vi "Find Intersecting Gaps.vi"(10 "Job Gaps Array":i32[][](array[numeric]), 11 "Machine Gaps Array":i32[][](array[numeric])) -> (3 "Gaps Array":T1[](array[typedef]))   [LabVIEW 2013, in "Scheduler.lvclass"]
uses:
  Scheduler.lvclass
  Controls/ValidGaps.ctl
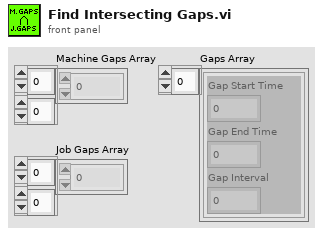
[diagram p1: front panel]
types:
  T1 = typedef "Scheduler.lvclass/ValidGaps.ctl" = cluster{"Gap Start Time":i32, "Gap End Time":i32, "Gap Interval":i32}
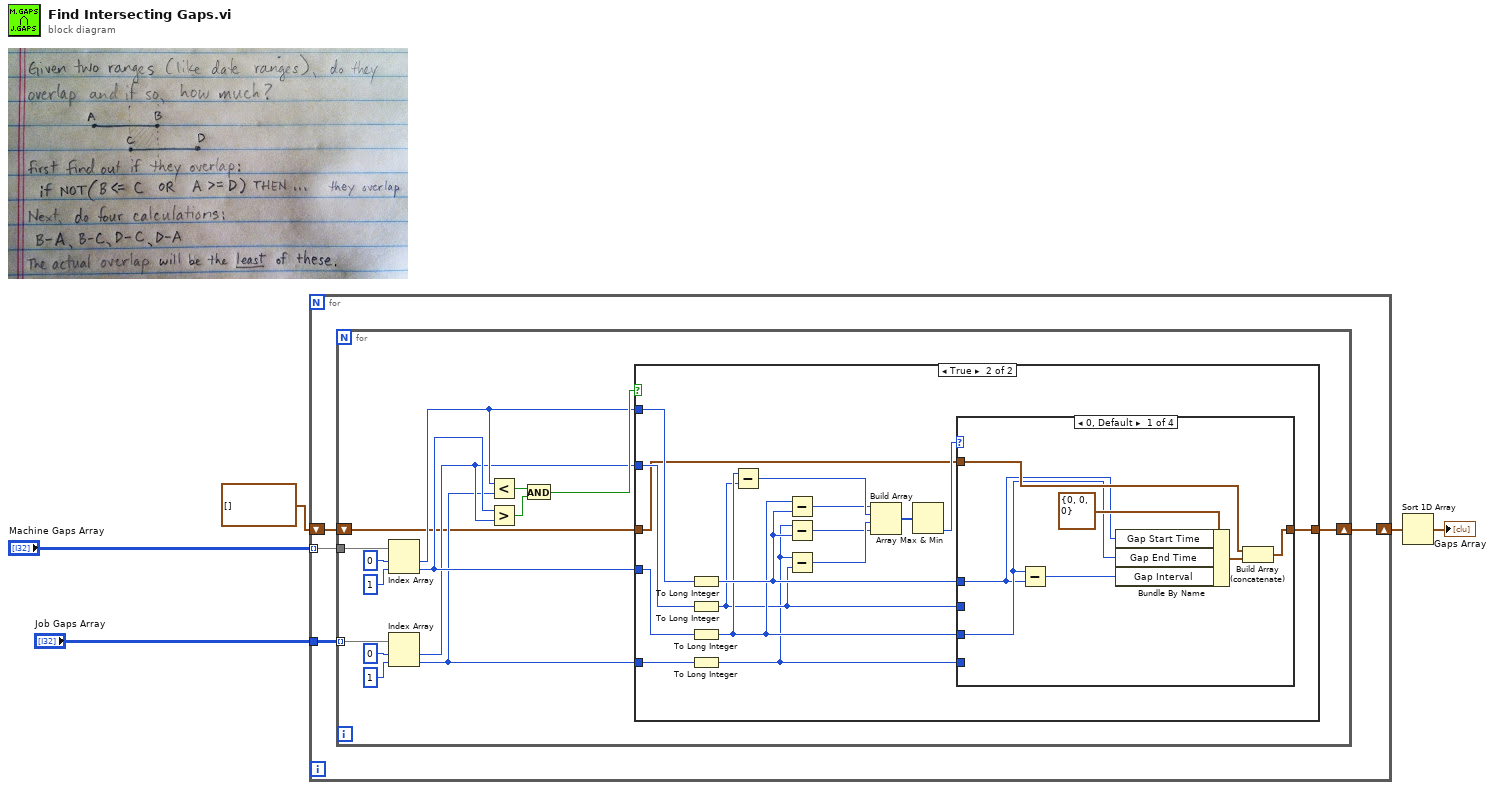
[diagram p0: block diagram]
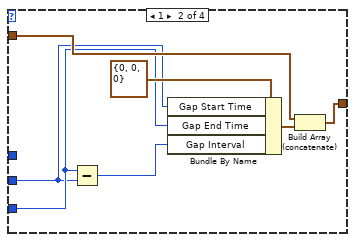
[diagram p3: hidden frame]
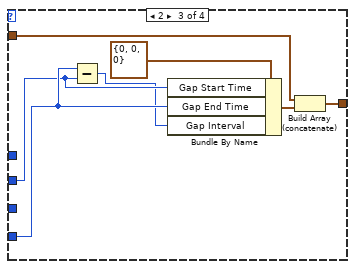
[diagram p4: hidden frame]
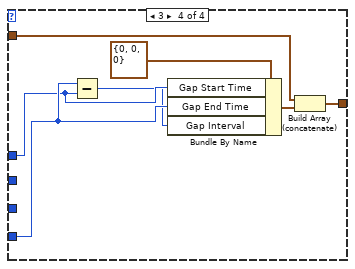
[diagram p5: hidden frame]
diagram:
  n1 = for {
    tunnel: "Machine Gaps Array" -> [w8] mode=indexing
    tunnel: "Job Gaps Array" -> [w9]
    shift-right: [w6] -> w1
    shift-left: T1[] [] -> [w7]
    n2 = for {
      tunnel: w9 -> [w24] mode=indexing
      tunnel: w8 -> [w21]
      shift-right: [w10] -> w6
      shift-left: w7 -> [w11]
      n3 = Index Array(array=w21, index #1=0 ("index"), index #2=1 ("index")) -> (element #1=w14:i32, element #2=w15:i32)
      n4 = Index Array(array=w24, index #1=0 ("index"), index #2=1 ("index")) -> (element #1=w13:i32, element #2=w12:i32)
      n5 = Less?(x=w14, y=w12) -> (x < y?=w18:bool)
      n6 = Greater?(x=w15, y=w13) -> (0:w17:bool)
      n7 = And(x=w18, y=w17) -> (x .and. y?=w16:bool)
      n8 = case shown="True" w16 {
        tunnel: w15 -> [_ w41]
        tunnel: w14 -> [_ w40]
        tunnel: w13 -> [_ w39]
        tunnel: w12 -> [_ w38]
        tunnel: w11 -> [w25 w27]
        tunnel: [w25 w26] -> w10
        frame False {
        }
        frame True {
          n9 = To Long Integer(number=w40) -> (32bit integer=w31:i32)
          n10 = To Long Integer(number=w39) -> (32bit integer=w29:i32)
          n11 = To Long Integer(number=w41) -> (32bit integer=w30:i32)
          n12 = To Long Integer(number=w38) -> (32bit integer=w28:i32)
          n13 = Subtract(x=w30, y=w29) -> (x-y=w37:i32)
          n14 = Subtract(x=w30, y=w31) -> (x-y=w32:i32)
          n15 = Subtract(x=w28, y=w31) -> (x-y=w35:i32)
          n16 = Subtract(x=w28, y=w29) -> (x-y=w36:i32)
          n17 = Build Array(w32, w37, w36, w35) -> (w34:i32[])
          n18 = Array Max & Min(array=w34) -> (min index (indices)=w33:i32)  [unwired: 3 out]
          n19 = case shown="0, Default" w33 {
            tunnel: w31 -> [w43 _ _ w64]
            tunnel: w30 -> [w44 w51 _ _]
            tunnel: w29 -> [_ w50 w57 _]
            tunnel: w28 -> [_ _ w58 w65]
            tunnel: w27 -> [w48 w55 w62 w69]
            tunnel: [w46 w53 w60 w67] -> w26
            frame 0, Default {
              n20 = Subtract(x=w44, y=w43) -> (x-y=w42:i32)
              n21 = Bundle By Name(cluster=T1 {"Gap Start Time"=0, "Gap End Time"=0, "Gap Interval"=0}, "Gap Start Time"=w43, "Gap End Time"=w44, "Gap Interval"=w42) -> (w47:T1)
              n22 = Build Array (concatenate)(w48, w47) -> (w46:T1[])
            }
            frame 1 {
              n23 = Subtract(x=w51, y=w50) -> (x-y=w49:i32)
              n24 = Bundle By Name(cluster=T1 {"Gap Start Time"=0, "Gap End Time"=0, "Gap Interval"=0}, "Gap Start Time"=w50, "Gap End Time"=w51, "Gap Interval"=w49) -> (w54:T1)
              n25 = Build Array (concatenate)(w55, w54) -> (w53:T1[])
            }
            frame 2 {
              n26 = Subtract(x=w58, y=w57) -> (x-y=w56:i32)
              n27 = Bundle By Name(cluster=T1 {"Gap Start Time"=0, "Gap End Time"=0, "Gap Interval"=0}, "Gap Start Time"=w57, "Gap End Time"=w58, "Gap Interval"=w56) -> (w61:T1)
              n28 = Build Array (concatenate)(w62, w61) -> (w60:T1[])
            }
            frame 3 {
              n29 = Subtract(x=w65, y=w64) -> (x-y=w63:i32)
              n30 = Bundle By Name(cluster=T1 {"Gap Start Time"=0, "Gap End Time"=0, "Gap Interval"=0}, "Gap Start Time"=w64, "Gap End Time"=w65, "Gap Interval"=w63) -> (w68:T1)
              n31 = Build Array (concatenate)(w69, w68) -> (w67:T1[])
            }
          }
        }
      }
    }
  }
  n32 = Sort 1D Array(array=w1) -> (sorted array=→"Gaps Array":T1[])
